vi "WSVCAP SHL Host TL RFFE Write.vi"(0 "RFFE Data Out":u8[][](array[numeric]) format="%.0x", 5 "Socket Mask":u16=1 format="%02x", 11 "error in":errorcluster, 13 "Log (T)":bool=TRUE) -> (15 "error out":errorcluster)   [LabVIEW 2012]
uses:
  Type Defs/WSVCAP SHL Function Enum.ctl
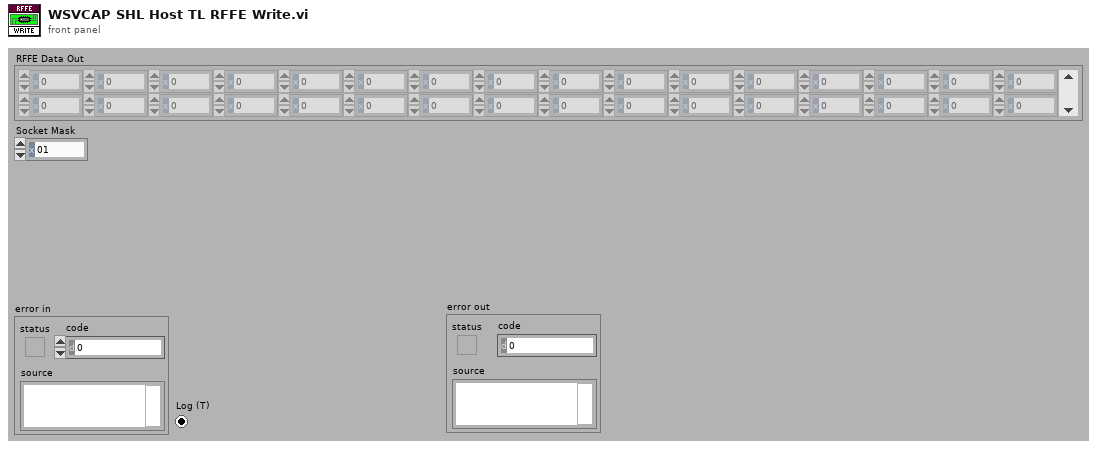
[diagram p1: front panel]
types:
  T1 = typedef "WSVCAP SHL Function Enum.ctl" = enum16{"Initialize", "Configure I2C", "Configure SPI", "Configure RFFE", "Write I2C", "Read I2C", "Write/Read SPI", "Start SPI Cycle", "Stop SPI Cycle", "Write RFFE", "Read RFFE", "Start RFFE Cycle", "Stop RFFE Cycle", "Get Status", "Close"}
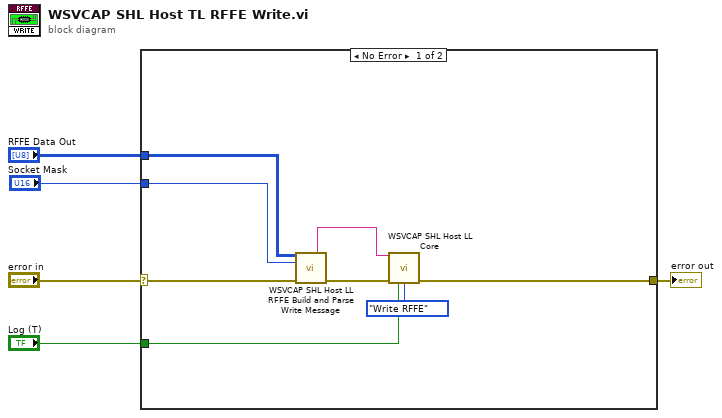
[diagram p0: block diagram]
diagram:
  n1 = case shown="No Error" "error in" {
    selector: "error in" -> [w10 w14]
    tunnel: [w6 w14] -> w5
    tunnel: "RFFE Data Out" -> [w9 _]
    tunnel: "Socket Mask" -> [w7 _]
    tunnel: "Log (T)" -> [w8 _]
    frame No Error {
      n2 = call "WSVCAP SHL Host LL RFFE Build and Parse Write Message.vi"("Write Data In [DUT Ordered]"=w9, "Socket Mask [U16] In"=w7, "error in"=w10) -> ("Message Out"=w11:string, "error out"=w12:errorcluster)  [unwired: 6 in, 5 out]
      n3 = call "WSVCAP SHL Host LL Core.vi"("Message In"=w11, "error in"=w12, "Log (T)"=w8, "Function"=WSVCAP_SHL_Function_Enum."Write RFFE") -> ("error out"=w6:errorcluster)  [unwired: 9 in, 2 out]
    }
    frame Error {
    }
  }
  "error out" <- w5
